vi "Fuzzy C-mean Clustering_de.vi"() -> ()   [LabVIEW 2010]
panel:
  in  "군집_데이터":i32[](array[numeric])
  in  "파일(대화 상자 사용)":path
  out "Array":ext[][](array[numeric])
  in  "cluster":i32=3
  out "Numeric":i32
  in  "임계값":ext=0.01
  out "Max":ext
  out "U0":ext[][](array[numeric])
  out "d":ext[][](array[numeric])
  out "v":ext[](array[numeric])
  out "n":i32
  out "j":i32
  out "U":ext[][](array[numeric])
  out "X":ext[][](array[numeric])
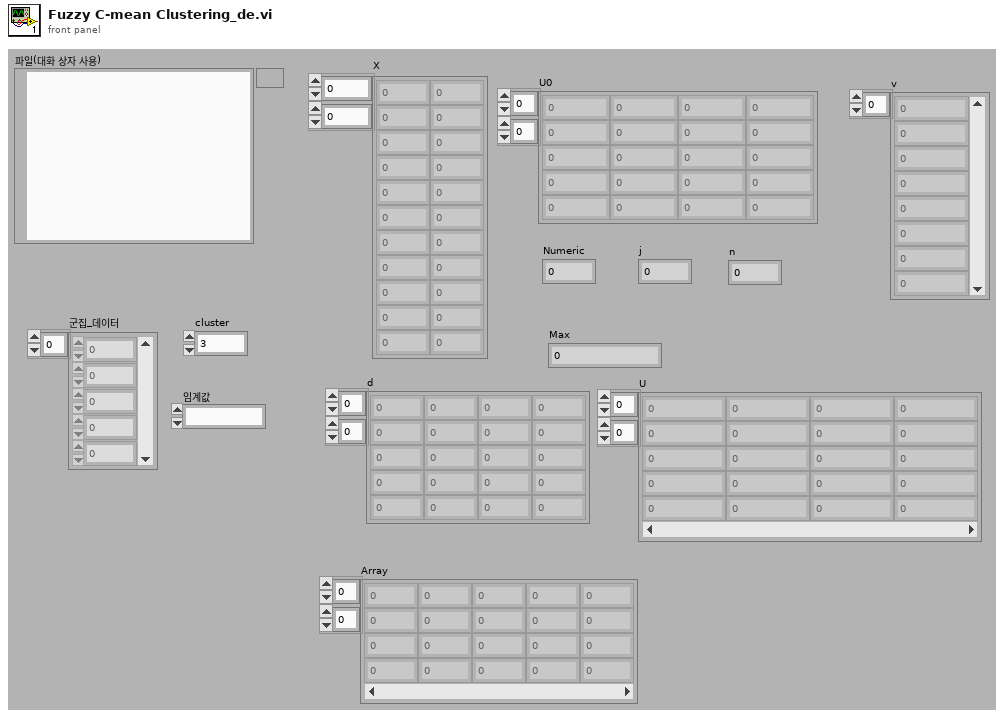
[diagram p1: front panel]
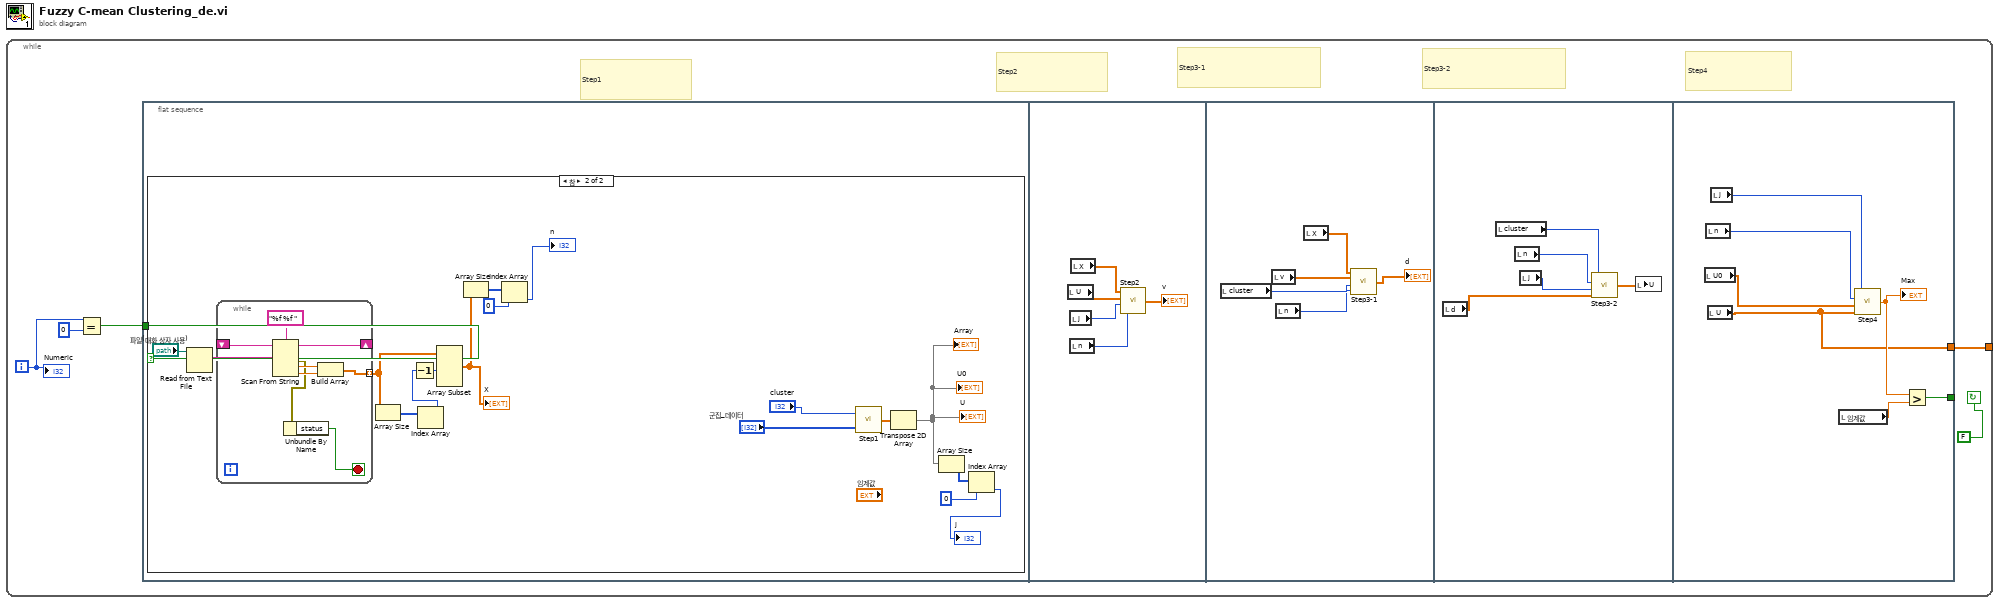
[diagram p0: block diagram]
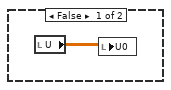
[diagram p2: hidden frame]
diagram:
  n1 = while {
    tunnel: [w2] -> _
    i -> [w5]
    stop <- FALSE continue-if-true
    # "Step4"
    # "Step3-2"
    # "Step3-1"
    # "Step2"
    # "Step1"
    n2 = Equal?(x=w5, y=0) -> (x = y?=w3:bool)
    n3 = flat-sequence {
      tunnel: w3 -> [w6]
      tunnel: [w50] -> _
      tunnel: [w48] -> w2
      frame #0 {
        n4 = case shown="참" w6 {
          frame False {
            n5 = local read "U"() -> (w7:ext[][])
            n6 = local write "U0"(w7) -> ()
          }
          frame True {
            n7 = Read from Text File(file (use dialog)="파일(대화 상자 사용)") -> (text=w20:string)  [unwired: 3 in, 3 out]
            n8 = while {
              shift-right: [w31] -> _
              shift-left: w20 -> [w32]
              tunnel: [w27] -> w24 mode=indexing
              stop <- w25 stop-if-true
              n9 = Scan From String(format string="%f %f " ("포맷 문자열"), input string=w32) -> (remaining string=w31:string, error out=w26:errorcluster, output 1=w29:dbl, output 2=w28:dbl)  [unwired: 4 in, 1 out]
              n10 = Unbundle By Name(w26) -> ("status"=w25:bool)
              n11 = Build Array(w29, w28) -> (w27:dbl[])
            }
            n12 = Array Size(array=w24) -> (size(s)=w21:i32[])
            n13 = Index Array(array=w21) -> (element=w22:i32)  [unwired: 1 in]
            n14 = Decrement(x=w22) -> (x-1=w23:i32)
            n15 = Array Subset(array=w24, length (row)=w23) -> (w14:dbl[][])  [unwired: 3 in]
            "X" <- w14
            n16 = Array Size(array=w14) -> (size(s)=w17:i32[])
            n17 = Index Array(array=w17, index=0) -> (element=→"n":i32)
            n18 = call "Step1.vi"("군집_데이터"="군집_데이터", "클러스터"="cluster") -> ("ALL_U"=w11:ext[][])
            n19 = Transpose 2D Array(2D array=w11) -> (transposed array=w8:ext[][])
            "U" <- w8
            "U0" <- w8
            "Array" <- w8
            n20 = Array Size(array=w8) -> (size(s)=w15:i32[])
            n21 = Index Array(array=w15, index=0) -> (element=→"j":i32)
          }
        }
      }
      frame #1 {
        n22 = local read "U"() -> (w35:ext[][])
        n23 = local read "j"() -> (w33:i32)
        n24 = local read "n"() -> (w34:i32)
        n25 = local read "X"() -> (w36:ext[][])
        n26 = call "Step2.vi"("n"=w34, "j"=w33, "U"=w35, "X"=w36) -> ("v"=→"v":dbl[])
      }
      frame #2 {
        n27 = local read "cluster"() -> (w42:i32)
        n28 = local read "v"() -> (w39:ext[])
        n29 = local read "n"() -> (w38:i32)
        n30 = local read "X"() -> (w40:ext[][])
        n31 = call "Step3-1.vi"("cluster"=w42, "n"=w38, "v"=w39, "X"=w40) -> ("Array"=→"d":dbl[][])
      }
      frame #3 {
        n32 = local read "d"() -> (w43:ext[][])
        n33 = local read "cluster"() -> (w46:i32)
        n34 = local read "n"() -> (w45:i32)
        n35 = local read "j"() -> (w44:i32)
        n36 = call "Step3-2.vi"("d"=w43, "j"=w44, "n"=w45, "cluster"=w46) -> ("Array"=w47:dbl[][])
        n37 = local write "U"(w47) -> ()
      }
      frame #4 {
        n38 = local read "U0"() -> (w53:ext[][])
        n39 = local read "n"() -> (w49:i32)
        n40 = local read "U"() -> (w48:ext[][])
        n41 = local read "j"() -> (w54:i32)
        n42 = local read "임계값"() -> (w51:ext)
        n43 = call "Step4.vi"("U"=w48, "U0"=w53, "n"=w49, "j"=w54) -> ("Numeric"=w52:dbl)
        "Max" <- w52
        n44 = Greater?(x=w52, y=w51) -> (0:w50:bool)
      }
    }
    "Numeric" <- w5
  }
